vi "Configure Control AI Range(Volt Scale).vi"(0 "VISA resource name":refnum<visa-resource-name>, 1 "Unit No. (0)":i32 min=0 max=6, 3 "Range And Span":T2={"Volt Range (4 : 2V)"=4, "Enable Span (False)"=FALSE, "Lower Span (2.0000)"=-2.0, "Upper Span (2.0000)"=2.0, "Bias (0)"=0.0} {"Upper Span (2.0000)" min=-99999.0 max=99999.0 step=1.0 format="%_5g"; "Lower Span (2.0000)" min=-99999.0 max=99999.0 step=1.0 format="%_5g"; "Volt Range (4 : 2V)" items=["20mV", "60mV", "200mV", "1V", "2V", "6V", "20V", "50V"]}, 4 "Module No.(0)":i32 min=0 max=9, 5 "AI No.(1)":i32=1 min=1 max=2, 7 "error in (no error)":errorcluster, 8 "Scaling":T1={"Floating Point Position (2)"=2, "Lower Scaling (0)"=0.0, "Upper Scaling (10000)"=100.0, "Unit Character (\"\")"=""} {"Upper Scaling (10000)" format="%_6g"; "Lower Scaling (0)" format="%_6g"; "Floating Point Position (2)" min=0 max=5 step=1}) -> (20 "VISA resource name out":refnum<visa-resource-name>, 21 "AI No.":i32, 24 "Unit No.":i32, 25 "Module No.":i32, 27 "error out":errorcluster)   [LabVIEW 2020, in "Yokogawa GX Series.lvlib"]
doc: "Set Volt range of AI channel in PID module.\n\nCommand: SCtrlRangeAI"
uses:
  <instrlib>/Yokogawa GX Series/Yokogawa GX Series.lvlib
  <instrlib>/Yokogawa GX Series/Private/Volt Range.vi
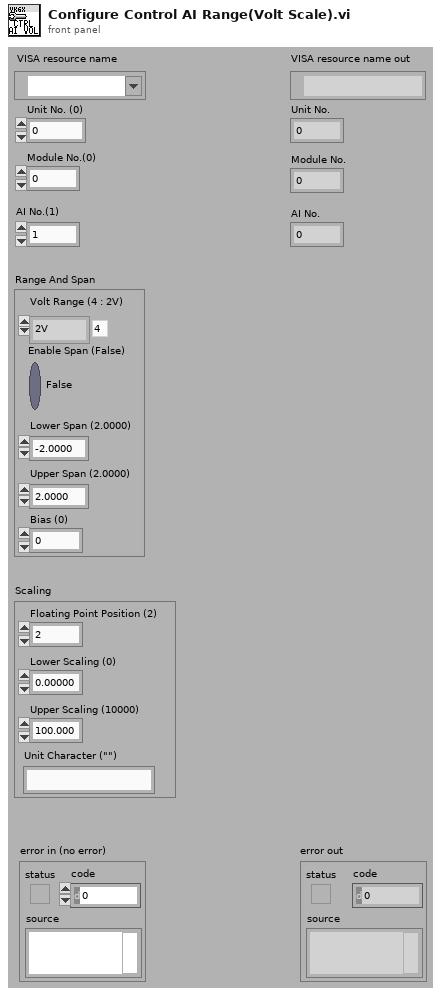
[diagram p1: front panel]
types:
  T1 = cluster{"Floating Point Position (2)":i32, "Lower Scaling (0)":dbl, "Upper Scaling (10000)":dbl, "Unit Character (\"\")":string}
  T2 = cluster{"Volt Range (4 : 2V)":i32, "Enable Span (False)":bool, "Lower Span (2.0000)":dbl, "Upper Span (2.0000)":dbl, "Bias (0)":dbl}
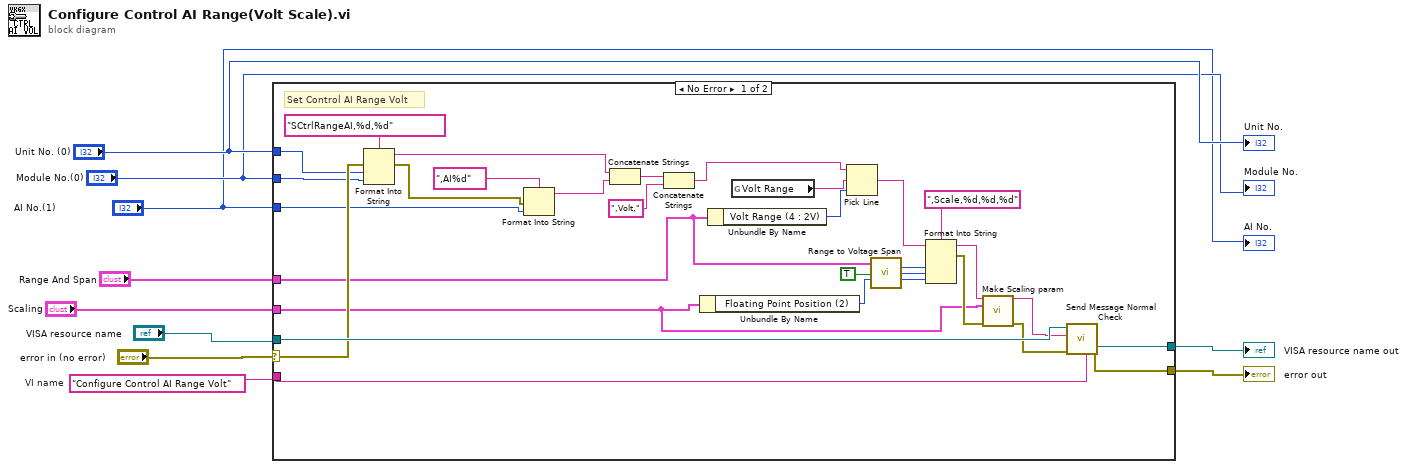
[diagram p0: block diagram]
diagram:
  w6 = "Configure Control AI Range Volt"  # VI name
  n1 = case shown="No Error" "error in (no error)" {
    selector: "error in (no error)" -> [w37 w42]
    tunnel: [w41 w43] -> w10
    tunnel: [w40 w42] -> w9
    tunnel: "VISA resource name" -> [w39 w43]
    tunnel: w6 -> [w36 _]
    tunnel: "Unit No. (0)" -> [w35 _]
    tunnel: "Module No.(0)" -> [w34 _]
    tunnel: "AI No.(1)" -> [w32 _]
    tunnel: "Range And Span" -> [w16 _]
    tunnel: "Scaling" -> [w13 _]
    frame No Error {
      # "Set Control AI Range Volt"
      n2 = Format Into String(format string="SCtrlRangeAI,%d,%d", error in=w37, w35, w34) -> (resulting string=w30:string, error out=w31:errorcluster)  [unwired: 1 in]
      n3 = Format Into String(format string=",AI%d", error in=w31, w32) -> (resulting string=w29:string)  [unwired: 1 in, 1 out]
      n4 = Concatenate Strings(w30, w29) -> (w28:string)
      n5 = Concatenate Strings(w28, ",Volt,") -> (w18:string)
      n6 = Unbundle By Name(w13) -> ("Floating Point Position (2)"=w20:i32)
      n7 = Unbundle By Name(w16) -> ("Volt Range (4 : 2V)"=w26:i32)
      n8 = global read "Volt Range.vi" "Volt Range"() -> (w17:string)
      n9 = Pick Line(string ("")=w18, multi-line string=w17, line index=w26) -> (output string=w15:string)
      n10 = call <instrlib>:"Range to Voltage Span.vi"("Range And Span"=w16, "Scaling? (False)"=TRUE, "Floating Point Position (2)"=w20) -> ("Lower Span"=w25:i32, "Upper Span"=w24:i32, "Bias"=w23:i32)  [unwired: 5 in, 5 out]
      n11 = Format Into String(format string=",Scale,%d,%d,%d", initial string=w15, w25, w24, w23) -> (resulting string=w19:string, error out=w21:errorcluster)  [unwired: 1 in]
      n12 = call <instrlib>:"Make Scaling param.vi"("String (\"\")"=w19, "Scaling"=w13, "error in (no error)"=w21) -> ("String After"=w12:string, "error out"=w11:errorcluster)  [unwired: 11 in]
      n13 = call <instrlib>:"Send Message Normal Check.vi"("Source (\"\")"=w36, "error in (no error)"=w11, "Send Message (\"\")"=w12, "VISA resource name"=w39) -> ("error out"=w40:errorcluster, "VISA resource name out"=w41:refnum<visa-resource-name>)  [unwired: 2 in, 4 out]
    }
    frame Error {
    }
  }
  "error out" <- w9
  "VISA resource name out" <- w10
  "Unit No." <- "Unit No. (0)"
  "Module No." <- "Module No.(0)"
  "AI No." <- "AI No.(1)"
